vi "NI VeriStand - Get Item Ref by Relative Path.vi"(8 "error in":errorcluster, 10 "Relative Item Path":string, 11 "Section Ref in":T1 format="%.0x") -> (0 "error out":errorcluster, 2 "Item Ref":T1 format="%.0x", 3 "Section Ref out":T1 format="%.0x", 4 "Found":bool)   [LabVIEW 2020, in "Custom Device Utility Library.lvlib"]
doc: "Returns a reference to a custom device item from a specified location relative to <B>Section Ref in</B>. Use one forward slash (/) as a separator between sections in the relative path. Like a standard file system, \"..\" traverses up the hierarchy one level. A leading forward slash indicates an absolute path from the root item of the hierarchy."
uses:
  <vilib>/NI VeriStand/Custom Device Tools/Custom Device Utility Library/Custom Device Utility Library.lvlib
  <vilib>/NI VeriStand/Custom Device API/Custom Device Item Ref.ctl
  <vilib>/NI VeriStand/Custom Device Tools/Custom Device Utility Library/NI VeriStand - Ref Constants.vi
  <vilib>/NI VeriStand/Custom Device API/Custom Device API.lvlib
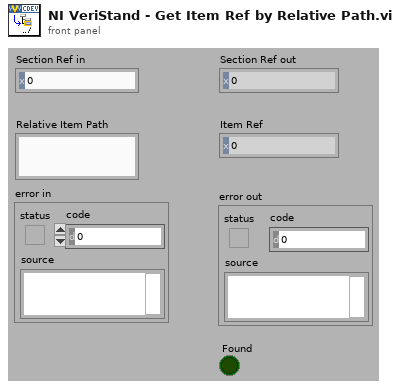
[diagram p1: front panel]
types:
  T1 = typedef "Custom Device API.lvlib/Custom Device Item Ref.ctl" = u64
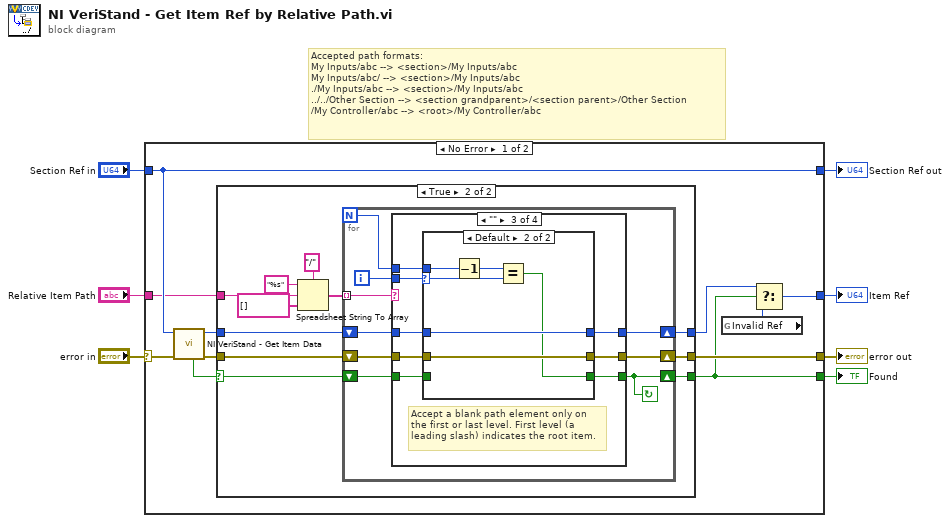
[diagram p0: block diagram]
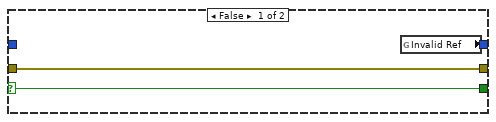
[diagram p2: hidden frame]
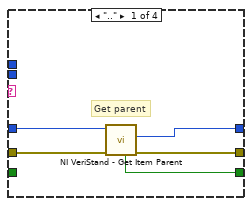
[diagram p3: hidden frame]
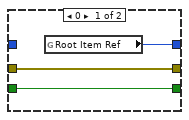
[diagram p5: hidden frame]
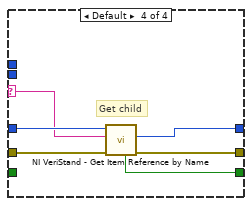
[diagram p6: hidden frame]
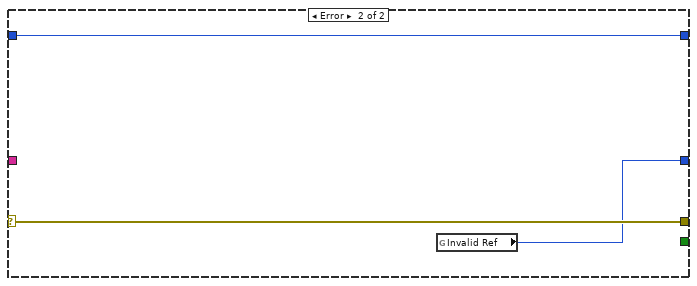
[diagram p7: hidden frame]
diagram:
  # "Accepted path formats:\nMy Inputs/abc --> <section>/My Inputs/abc\nMy Inputs/abc/ --> <section>/My Inputs/abc\n./My Inputs/abc --> <section>/My Inputs/abc\n../../Other Section --> <section grandparent>/<section parent>/Other Section\n/My Controller/abc --> <root>/My Controller/abc"
  n1 = case shown="No Error" "error in" {
    selector: "error in" -> [w12 w75]
    tunnel: [w10 _] -> w7
    tunnel: "Relative Item Path" -> [w16 _]
    tunnel: [w15 w75] -> w5
    tunnel: [w8 w73] -> w4
    tunnel: "Section Ref in" -> [w17 w74]
    tunnel: [w17 w74] -> w1
    frame No Error {
      n2 = call <vilib>:"NI VeriStand - Get Item Data.vi"("error in (no error)"=w12, "Item Ref in"=w17) -> ("error out"=w14:errorcluster, "Item Ref out"=w13:T1, "Found"=w11:bool)  [unwired: 7 out]
      n3 = case shown="True" w11 {
        selector: w11 -> [w21 w22]
        tunnel: [w21 w32] -> w10
        tunnel: w16 -> [_ w27]
        tunnel: [w20 w26] -> w15
        tunnel: [w19 w25] -> w9
        tunnel: w14 -> [w20 w24]
        tunnel: w13 -> [_ w23]
        frame False {
          n4 = global read "NI VeriStand - Ref Constants.vi" "Invalid Ref"() -> (w19:T1)
        }
        frame True {
          n5 = Spreadsheet String To Array(delimiter (Tab)="/", format string="%s", spreadsheet string=w27, array type (2D Dbl)=string[] []) -> (array=w31:string[])
          n6 = for {
            N -> [w34]
            shift-right: [w39] -> w25
            shift-left: w23 -> [w40]
            tunnel: w31 -> [w36] mode=indexing
            shift-right: [w38] -> w26
            shift-left: w24 -> [w41]
            shift-right: [w37] -> w32
            shift-left: w22 -> [w33]
            i -> [w35]
            stop <- w37 continue-if-true
            n7 = case shown="\"\"" w36 {
              tunnel: w41 -> [w46 w49 w57 w72]
              tunnel: w40 -> [w45 w48 w51 w71]
              tunnel: [w44 w48 w54 w70] -> w39
              tunnel: [w43 w49 w56 w69] -> w38
              tunnel: [w42 w47 w52 w68] -> w37
              tunnel: w35 -> [_ _ w55 _]
              tunnel: w34 -> [_ _ w50 _]
              tunnel: w33 -> [_ w47 w53 _]
              selector: w36 -> [_ _ _ w67]
              frame ".." {
                # "Get parent"
                n8 = call <vilib>:"NI VeriStand - Get Item Parent.vi"("error in (no error)"=w46, "Item Ref in"=w45) -> ("error out"=w43:errorcluster, "Parent Ref"=w44:T1, "Found"=w42:bool)  [unwired: 7 out]
              }
              frame "." {
                # "Stay at the current level."
              }
              frame "" {
                # "Accept a blank path element only on the first or last level. First level (a leading slash) indicates the root item."
                n9 = case shown="Default" w55 {
                  selector: w55 -> [_ w62]
                  tunnel: w57 -> [w59 w66]
                  tunnel: [w59 w66] -> w56
                  tunnel: [w60 w64] -> w54
                  tunnel: w53 -> [w58 _]
                  tunnel: [w58 w61] -> w52
                  tunnel: w51 -> [_ w64]
                  tunnel: w50 -> [_ w63]
                  frame 0 {
                    n10 = global read "NI VeriStand - Ref Constants.vi" "Root Item Ref"() -> (w60:T1)
                  }
                  frame Default {
                    n11 = Decrement(x=w63) -> (x-1=w65:i32)
                    n12 = Equal?(x=w65, y=w62) -> (x = y?=w61:bool)
                  }
                }
              }
              frame Default {
                # "Get child"
                n13 = call <vilib>:"NI VeriStand - Get Item Reference by Name.vi"("error in (no error)"=w72, "Item Name"=w67, "Parent Ref in"=w71) -> ("error out"=w69:errorcluster, "Item Ref"=w70:T1, "Found"=w68:bool)  [unwired: 6 out]
              }
            }
          }
        }
      }
      n14 = global read "NI VeriStand - Ref Constants.vi" "Invalid Ref"() -> (w18:T1)
      n15 = Select(t=w9, s=w10, f=w18) -> (s? t:f=w8:T1)
    }
    frame Error {
      n16 = global read "NI VeriStand - Ref Constants.vi" "Invalid Ref"() -> (w73:T1)
    }
  }
  "Found" <- w7
  "error out" <- w5
  "Section Ref out" <- w1
  "Item Ref" <- w4
